vi "Assign switches.vi"(1 "Array":T2(array[cluster])=[{"Channel x"="x6", "Channel y"="y1"}, {"Channel x"="x2", "Channel y"="y5"}]) -> (0 "Array 2":T1(array[cluster])=[{"result string"="xA6", "result string"="yA1"}, {"result string"="comB6", "result string"="chB6"}, {"result string"="comD1", "result string"="chD1"}, {"result string"="xA2", "result string"="yA5"}, {"result string"="comC2", "result string"="chC2"}, {"result string"="comD5", "result string"="chD5"}])   [LabVIEW 2011]
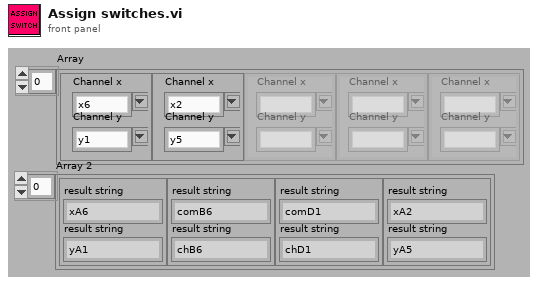
[diagram p1: front panel]
types:
  T1 = cluster{"result string":string, "result string":string}[]
  T2 = cluster{"Channel x":string, "Channel y":string}[]
  T3 = cluster{"result string":string, "result string":string}
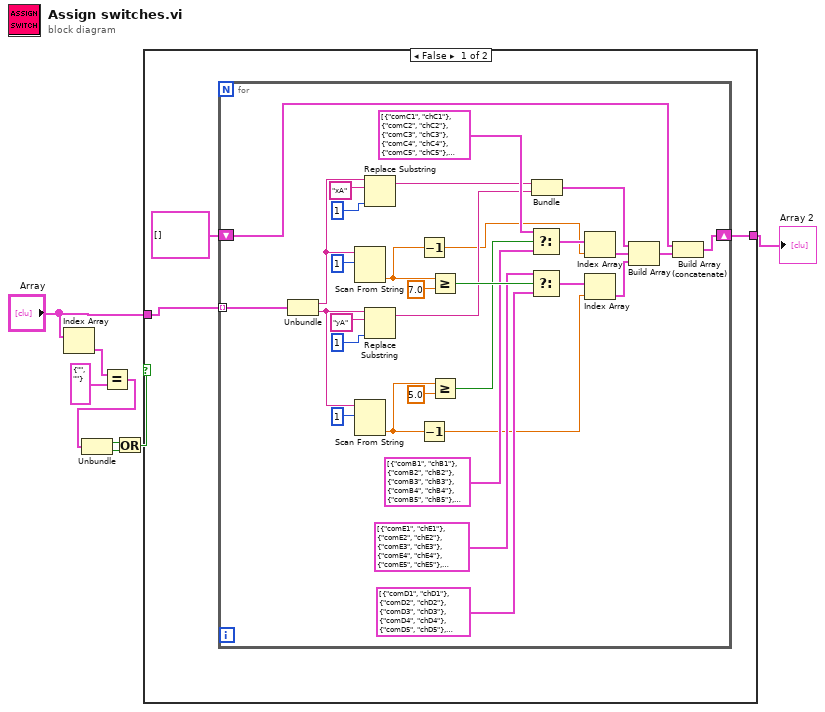
[diagram p0: block diagram]
diagram:
  n1 = Index Array(array="Array") -> (element=w6:cluster{"Channel x":string, "Channel y":string})  [unwired: 1 in]
  n2 = Equal?(x=w6, y=cluster{"Channel x":string, "Channel y":string} {"Channel x"="", "Channel y"=""}) -> (x = y?=w4:cluster{"Channel x":bool, "Channel y":bool})
  n3 = Unbundle(w4) -> ("Channel x"=w3:bool, "Channel y"=w2:bool)
  n4 = Or(x=w3, y=w2) -> (x .or. y?=w1:bool)
  n5 = case shown="False" w1 {
    tunnel: "Array" -> [w9 w43]
    tunnel: [w10 w43] -> w8
    frame False {
      n6 = for {
        tunnel: w9 -> [w12] mode=indexing
        shift-right: [w14] -> w10
        shift-left: T1 [] -> [w13]
        n7 = Unbundle(w12) -> ("Channel x"=w17:string, "Channel y"=w16:string)
        n8 = Scan From String(input string=w17, initial scan location=u32 1) -> (output 1=w27:dbl)  [unwired: 3 in, 3 out]
        n9 = Scan From String(input string=w16, initial scan location=u32 1) -> (output 1=w25:dbl)  [unwired: 3 in, 3 out]
        n10 = Replace Substring(2:1 ("length (len. of substring)"), 4:"xA" ("substring (\"\")"), 5:w17) -> (1:w24:string)  [unwired: 1 in, 1 out]
        n11 = Replace Substring(2:1 ("length (len. of substring)"), 4:"yA" ("substring (\"\")"), 5:w16) -> (1:w23:string)  [unwired: 1 in, 1 out]
        n12 = Decrement(x=w27) -> (x-1=w20:dbl)
        n13 = Decrement(x=w25) -> (x-1=w21:dbl)
        n14 = Greater Or Equal?(x=w27, y=7.0) -> (x >= y?=w38:bool)
        n15 = Greater Or Equal?(x=w25, y=5.0) -> (x >= y?=w37:bool)
        n16 = Select(t=cluster{string, string}[] [{"comC1", "chC1"}, {"comC2", "chC2"}, {"comC3", "chC3"}, {"comC4", "chC4"}, {"comC5", "chC5"}, {"comC6", "chC6"}, {"comC7", "chC7"}, {"comC8", "chC8"}, {"comC9", "chC9"}, {"comC10", "chC10"}, {"comC11", "chC11"}, {"comC12", "chC12"}] ("Switch C"), s=w37, f=cluster{string, string}[] [{"comB1", "chB1"}, {"comB2", "chB2"}, {"comB3", "chB3"}, {"comB4", "chB4"}, {"comB5", "chB5"}, {"comB6", "chB6"}, {"comB7", "chB7"}, {"comB8", "chB8"}, {"comB9", "chB9"}, {"comB10", "chB10"}, {"comB11", "chB11"}, {"comB12", "chB12"}] ("Switch B")) -> (s? t:f=w26:cluster{string, string}[])
        n17 = Select(t=cluster{string, string}[] [{"comE1", "chE1"}, {"comE2", "chE2"}, {"comE3", "chE3"}, {"comE4", "chE4"}, {"comE5", "chE5"}, {"comE6", "chE6"}, {"comE7", "chE7"}, {"comE8", "chE8"}] ("Switch E"), s=w38, f=cluster{string, string}[] [{"comD1", "chD1"}, {"comD2", "chD2"}, {"comD3", "chD3"}, {"comD4", "chD4"}, {"comD5", "chD5"}, {"comD6", "chD6"}, {"comD7", "chD7"}, {"comD8", "chD8"}] ("Switch D")) -> (s? t:f=w28:cluster{string, string}[])
        n18 = Bundle("result string"=w24, "result string"=w23) -> (w22:T3)  [unwired: 1 in]
        n19 = Index Array(array=w26, index=w20) -> (element=w18:cluster{string, string})
        n20 = Index Array(array=w28, index=w21) -> (element=w19:cluster{string, string})
        n21 = Build Array(w22, w18, w19) -> (w15:T1)
        n22 = Build Array (concatenate)(w13, w15) -> (w14:T1)
      }
    }
    frame True {
    }
  }
  "Array 2" <- w8
